vi "checkBeginPreparePenaltyAllyPlayVSS.vi"(8 "error in (no error)":errorcluster, 9 "last command_interpreted":T1, 10 "Game":refnum<class "Game.lvclass">, 11 "PreparePenaltyAllyPlayVSS in":refnum<class "PreparePenaltyAllyPlayVSS.lvclass">) -> (0 "error out":errorcluster, 2 "Boolean":bool, 3 "PreparePenaltyAllyPlayVSS out":refnum<class "PreparePenaltyAllyPlayVSS.lvclass">)   [LabVIEW 2018, in "PreparePenaltyAllyPlayVSS.lvclass"]
uses:
  PreparePenaltyAllyPlayVSS.lvclass
  Game_class/Game.lvclass
  Referee_class/command_interpreted.ctl
  Game_class/Game.lvclass/Game.ctl
  Referee_class/Referee.lvclass/Referee.ctl
  Game_class/Read Referee.vi
  Referee_class/Read command_interpreted.vi
  Referee_class/Referee.lvclass
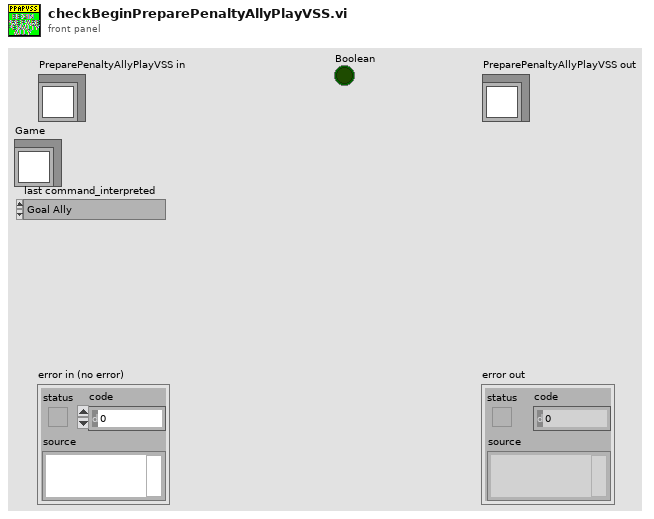
[diagram p1: front panel]
types:
  T1 = typedef "command_interpreted.ctl" = enum16{"Goal Ally", "Goal Enemy", "Ball Placement Enemy", "Ball Placement Ally", "Normal Half Time", "Extra Time  Break", "Extra Half Time", "None", "Post Game", "PKA Normal Start", "Prepare Kickoff Ally", "PKE Normal Start", "Prepare Kickoff Enemy", "Force Start", "Halt", "Timeout", "Prepare Penalty Ally", "Prepare Penalty Enemy", "PPA NormalStart", "PPE Normal Start", "Indirect Free Ally", "Direct Free Enemy", "Direct Free Ally", "Indirect Free Enemy", "Stop"}
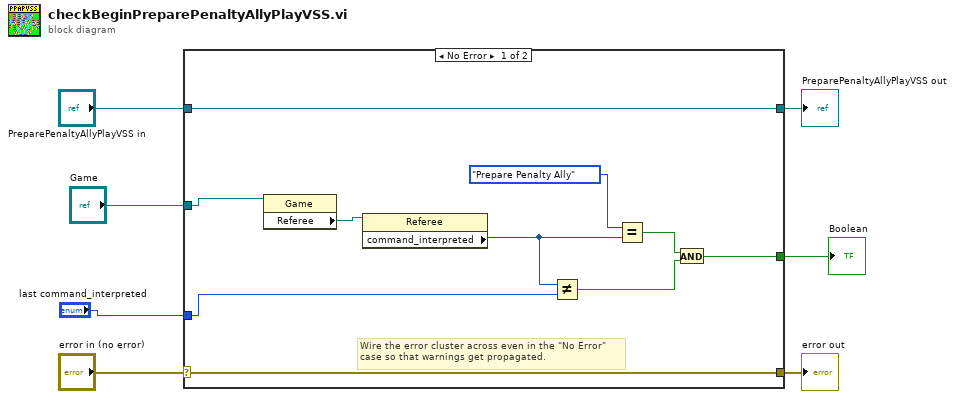
[diagram p0: block diagram]
diagram:
  n1 = case shown="No Error" "error in (no error)" {
    selector: "error in (no error)" -> [w16 w19]
    tunnel: [w16 w19] -> w6
    tunnel: [w17 w18] -> w4
    tunnel: "PreparePenaltyAllyPlayVSS in" -> [w17 w18]
    tunnel: "Game" -> [w15 _]
    tunnel: "last command_interpreted" -> [w11 _]
    tunnel: [w8 _] -> w1
    frame No Error {
      # "Wire the error cluster across even in the \"No Error\"\ncase so that warnings get propagated."
      n2 = property class="Game"(reference=w15) -> ("Referee"=w14:refnum<class "Referee.lvclass">)  [unwired: 1 in, 2 out]
      n3 = property class="Referee"(reference=w14) -> ("command_interpreted"=w12:T1)  [unwired: 1 in, 2 out]
      n4 = Not Equal?(x=w12, y=w11) -> (x != y?=w9:bool)
      n5 = Equal?(x=command_interpreted."Prepare Penalty Ally" ("command_interpreted"), y=w12) -> (x = y?=w10:bool)
      n6 = And(x=w10, y=w9) -> (x .and. y?=w8:bool)
    }
    frame Error {
    }
  }
  "error out" <- w6
  "PreparePenaltyAllyPlayVSS out" <- w4
  "Boolean" <- w1
